vi "Sort Corners.vi"(10 "Rectangle Descriptor 2":T1) -> (2 "output cluster":T1)   [LabVIEW 2025]
uses:
  8ab0638f-228f-4cc2-a02c-1e499da2c410.vi
  <vilib>/Array/Sort 2D Array - Pop Stack.vi
  <vilib>/Array/Sort 2D Array - Push Stack.vi
  8ab0638f-228f-4cc2-a02c-1e499da2c410.vi/269d4b3b-47f5-49e3-8884-44851e4dd9d5.vi
  8ab0638f-228f-4cc2-a02c-1e499da2c410.vi/6d99389c-673d-4efb-bf33-19b32bcf4cf8.vi
panel:
  out "sorted 2D array":sgl[][](array[numeric])
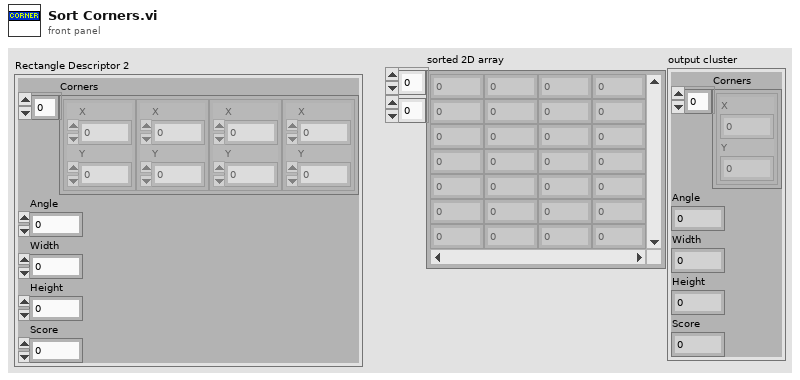
[diagram p1: front panel]
types:
  T1 = cluster{"Corners":cluster{"X":sgl, "Y":sgl}[], "Angle":dbl, "Width":dbl, "Height":dbl, "Score":dbl}
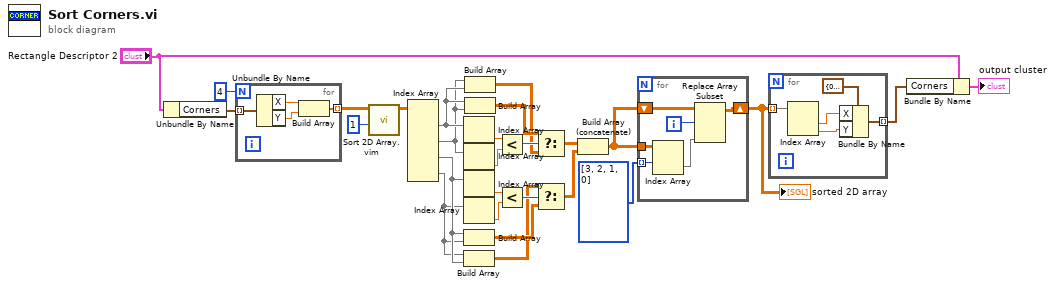
[diagram p0: block diagram]
diagram:
  n1 = Unbundle By Name("Rectangle Descriptor 2") -> ("Corners"=w24:cluster{"X":sgl, "Y":sgl}[])
  n2 = for {
    N: 4 -> [_]
    tunnel: w24 -> [w31] mode=indexing
    tunnel: [w28] -> w26 mode=indexing
    n3 = Unbundle By Name(w31) -> ("X"=w30:sgl, "Y"=w29:sgl)
    n4 = Build Array(w30, w29) -> (w28:sgl[])
  }
  n5 = call "Sort 2D Array.vim"("index"=1, "2D array"=w26) -> ("sorted 2D array"=w21:sgl[][])  [unwired: 8 in, 1 out]
  n6 = Index Array(array=w21) -> (element #1=w14:sgl[], element #2=w13:sgl[], element #3=w9:sgl[], element #4=w8:sgl[])  [unwired: 8 in]
  n7 = Index Array(array=w14) -> (element=w20:sgl)  [unwired: 1 in]
  n8 = Index Array(array=w13) -> (element=w19:sgl)  [unwired: 1 in]
  n9 = Index Array(array=w9) -> (element=w17:sgl)  [unwired: 1 in]
  n10 = Index Array(array=w8) -> (element=w18:sgl)  [unwired: 1 in]
  n11 = Build Array(w9, w8) -> (w6:sgl[][])
  n12 = Build Array(w8, w9) -> (w5:sgl[][])
  n13 = Build Array(w13, w14) -> (w12:sgl[][])
  n14 = Build Array(w14, w13) -> (w15:sgl[][])
  n15 = Less?(x=w20, y=w19) -> (x < y?=w16:bool)
  n16 = Less?(x=w17, y=w18) -> (x < y?=w10:bool)
  n17 = Select(t=w15, s=w16, f=w12) -> (s? t:f=w11:sgl[][])
  n18 = Select(t=w5, s=w10, f=w6) -> (s? t:f=w7:sgl[][])
  n19 = Build Array (concatenate)(w11, w7) -> (w2:sgl[][])
  n20 = for {
    shift-right: [w36] -> w3
    shift-left: w2 -> [w37]
    tunnel: w2 -> [w34]
    tunnel: i32[] [3, 2, 1, 0] -> [w33] mode=indexing
    i -> [w35]
    n21 = Index Array(array=w34, index (row)=w33) -> (element=w32:sgl[])  [unwired: 1 in]
    n22 = Replace Array Subset(array=w37, new element=w32, index (row)=w35) -> (w36:sgl[][])  [unwired: 1 in]
  }
  "sorted 2D array" <- w3
  n23 = for {
    tunnel: w3 -> [w41] mode=indexing
    tunnel: [w38] -> w4 mode=indexing
    n24 = Index Array(array=w41) -> (element #1=w40:sgl, element #2=w39:sgl)  [unwired: 2 in]
    n25 = Bundle By Name(cluster=cluster{"X":sgl, "Y":sgl} {"X"=0.0, "Y"=0.0} ("Position"), "X"=w40, "Y"=w39) -> (w38:cluster{"X":sgl, "Y":sgl})
  }
  n26 = Bundle By Name(cluster="Rectangle Descriptor 2", "Corners"=w4) -> (→"output cluster":T1)
